vi "InitializeTirfLockedQueue.vi"(8 "error in (no error)":errorcluster, 10 "max queue size (-1, unlimited)":i32=20, 11 "DAQ_QPT_Throlab in":refnum<class "DAQ_QPT_Throlab.lvclass">) -> (0 "error out":errorcluster, 3 "DAQ_QPT_Throlab out":refnum<class "DAQ_QPT_Throlab.lvclass">)   [LabVIEW 2020, in "DAQ_QPT_Throlab.lvlib" / "DAQ_QPT_Throlab.lvclass"]
uses:
  DAQ_QPT_Throlab.lvclass
  DAQ_QPT_Throlab.lvclass/DAQ_QPT_Throlab.ctl
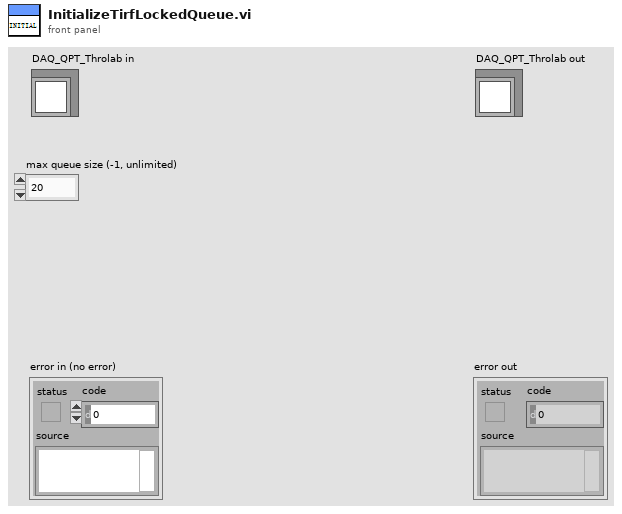
[diagram p1: front panel]
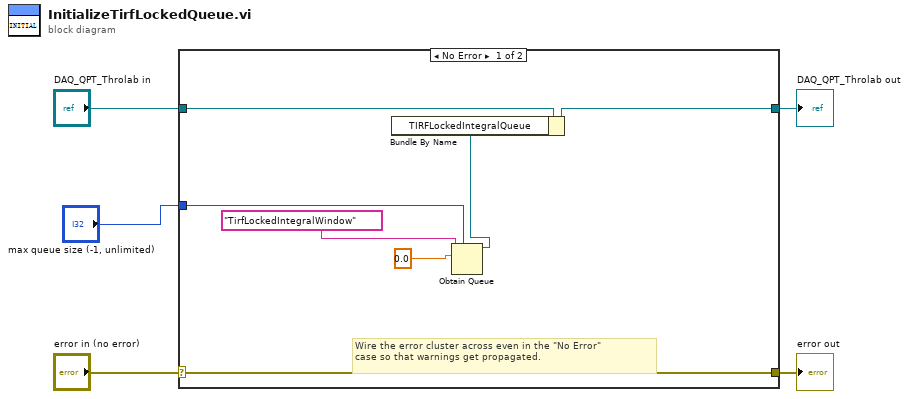
[diagram p0: block diagram]
diagram:
  n1 = case shown="No Error" "error in (no error)" {
    selector: "error in (no error)" -> [w11 w14]
    tunnel: [w11 w14] -> w4
    tunnel: [w8 w13] -> w2
    tunnel: "DAQ_QPT_Throlab in" -> [w12 w13]
    tunnel: "max queue size (-1, unlimited)" -> [w6 _]
    frame No Error {
      # "Wire the error cluster across even in the \"No Error\"\ncase so that warnings get propagated."
      n2 = Obtain Queue(max queue size (-1, unlimited)=w6, name (unnamed)="TirfLockedIntegralWindow", element data type=0.0 ("Interval(ms)")) -> (queue out=w7:refnum<queue>)  [unwired: 2 in, 2 out]
      n3 = Bundle By Name(cluster=w12, "TIRFLockedIntegralQueue"=w7) -> (w8:refnum<class "DAQ_QPT_Throlab.lvclass">)
    }
    frame Error {
    }
  }
  "error out" <- w4
  "DAQ_QPT_Throlab out" <- w2
